vi "Create Notifiers.vi"(8 "error in":errorcluster) -> (0 "error out":errorcluster, 3 "Notifiers":T1)   [LabVIEW 2014, in "Notifiers.lvlib"]
doc: "Creates notifiers for handshaking and closing processes"
uses:
  Notifiers.lvlib
  Notifiers.ctl
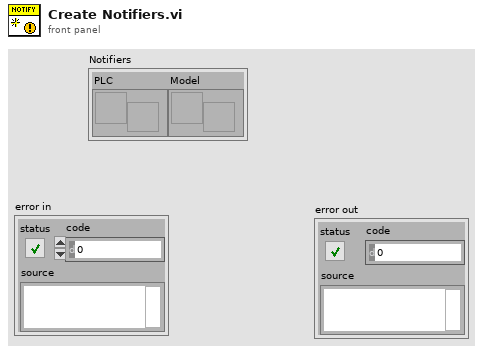
[diagram p1: front panel]
types:
  T1 = typedef "Notifiers.lvlib/Notifiers.ctl" = cluster{"PLC":refnum<notifier>, "Model":refnum<notifier>}
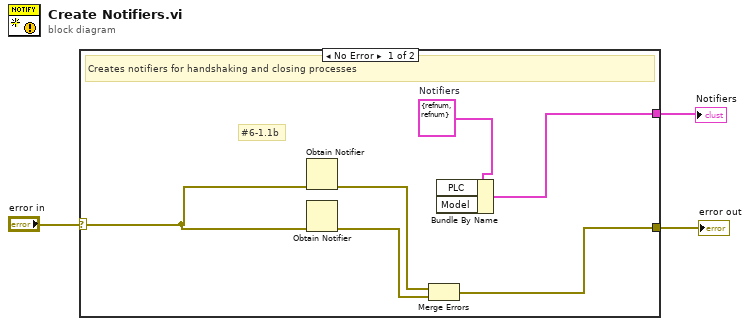
[diagram p0: block diagram]
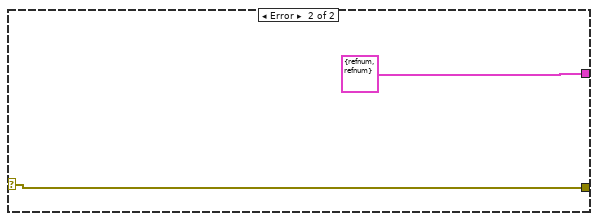
[diagram p2: hidden frame]
diagram:
  n1 = case shown="No Error" "error in" {
    selector: "error in" -> [w5 w11]
    tunnel: [w8 w11] -> w3
    tunnel: [w7 T1 {"PLC"=refnum, "Model"=refnum} ("Notifiers")] -> w2
    frame No Error {
      w4 = T1 {"PLC"=refnum, "Model"=refnum}  # Notifiers
      # "#6-1.1b"
      # "Creates notifiers for handshaking and closing processes"
      n2 = Obtain Notifier(error in (no error)=w5) -> (error out=w9:errorcluster)  [unwired: 3 in, 2 out]
      n3 = Obtain Notifier(error in (no error)=w5) -> (error out=w6:errorcluster)  [unwired: 3 in, 2 out]
      n4 = Merge Errors(w9, w6) -> (w8:errorcluster)
      n5 = Bundle By Name(cluster=w4) -> (w7:T1)  [unwired: 2 in]
    }
    frame Error {
    }
  }
  "error out" <- w3
  "Notifiers" <- w2
